vi "Auton - Drive Forward and Turn.vi"(11 "Auton States":T1=enum."Drive Forward") -> ()   [LabVIEW 2016]
uses:
  Auton - Drive Forward and Turn States.ctl
panel:
  in  "Setpoint":dbl=270.0 format="%#_13g"
  in  "Droven Forward?":bool
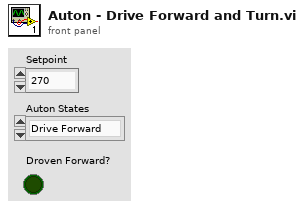
[diagram p1: front panel]
types:
  T1 = typedef "Auton - Drive Forward and Turn States.ctl" = enum16{"Stop", "Drive Forward", "Turn Left"}
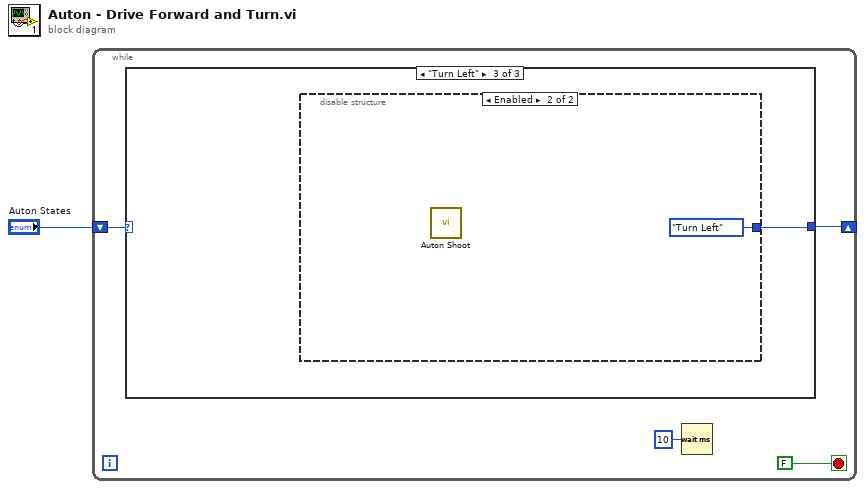
[diagram p0: block diagram]
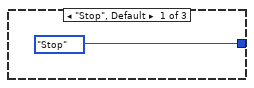
[diagram p2: hidden frame]
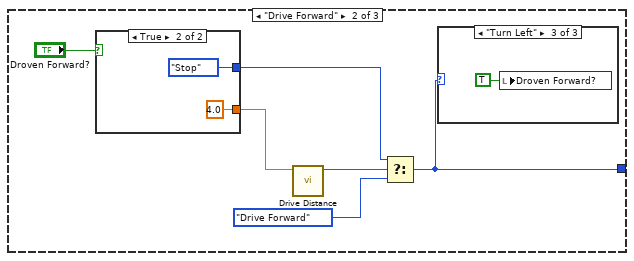
[diagram p3: hidden frame]
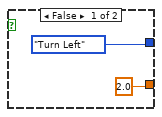
[diagram p6: hidden frame]
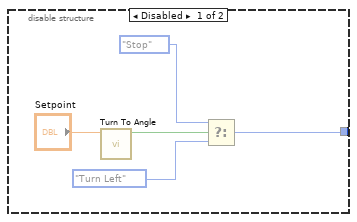
[diagram p7: hidden frame]
diagram:
  n1 = while {
    shift-right: [w4] -> _
    shift-left: "Auton States" -> [w5]
    stop <- FALSE stop-if-true
    n2 = case shown="\"Turn Left\"" w5 {
      tunnel: [Auton_-_Drive_Forward_and_Turn_States."Stop" ("Auton States") w7 w18] -> w4
      frame "Stop", Default {
      }
      frame "Drive Forward" {
        n3 = case shown="True" "Droven Forward?" {
          tunnel: [Auton_-_Drive_Forward_and_Turn_States."Turn Left" ("Auton States") Auton_-_Drive_Forward_and_Turn_States."Stop" ("Auton States")] -> w10
          tunnel: [2.0 ("Desired Distance") 4.0 ("Desired Distance")] -> w8
          frame False {
          }
          frame True {
          }
        }
        n4 = call "Drive Distance.vi"("Desired Distance"=w8) -> ("Done?"=w12:bool)  [unwired: 10 in]
        n5 = Select(t=w10, s=w12, f=Auton_-_Drive_Forward_and_Turn_States."Drive Forward" ("Auton States")) -> (s? t:f=w7:T1)
        n6 = case shown="\"Turn Left\"" w7 {
          frame "Stop", Default {
          }
          frame "Drive Forward" {
          }
          frame "Turn Left" {
            n7 = local write "Droven Forward?"(TRUE ("Droven Forward?")) -> ()
          }
        }
      }
      frame "Turn Left" {
        n8 = disable-structure shown="Enabled" {
          disable-tunnel: [w19 Auton_-_Drive_Forward_and_Turn_States."Turn Left" ("Auton States")] -> w18
          frame Disabled {
            n9 = call "Turn To Angle.vi"("Setpoint"="Setpoint") -> ("Done?"=w22:bool)  [unwired: 10 in]
            n10 = Select(t=Auton_-_Drive_Forward_and_Turn_States."Stop" ("Auton States"), s=w22, f=Auton_-_Drive_Forward_and_Turn_States."Turn Left" ("Auton States")) -> (s? t:f=w19:T1)
          }
          frame Enabled {
            n11 = call "Auton Shoot.vi"() -> ()  [unwired: 12 in]
          }
        }
      }
    }
    n12 = Wait (ms)(milliseconds to wait=u32 10) -> ()  [unwired: 1 out]
  }
